vi "Probe.vi"() -> ()   [LabVIEW 2020]
uses:
  source/PV Data/NT Base/NT Base.lvclass
  source/Client/Subscription/Subscription.lvclass
  source/Client/Client/Client.lvclass
  source/PV Data/Is Probeable/Is Probeable.lvclass
  source/Client/Subscription/Next Value - NT.vi
panel:
  in  "Search":bool
  in  "PV name":string
  in  "stop":bool
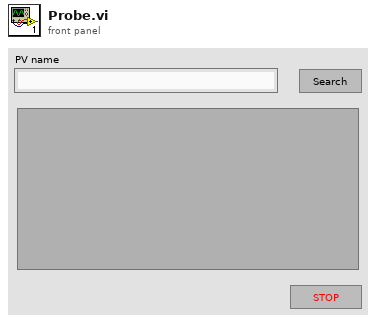
[diagram p1: front panel]
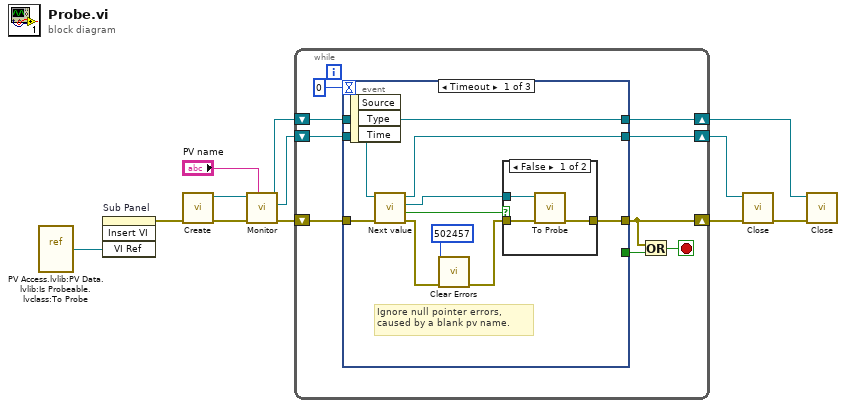
[diagram p0: block diagram]
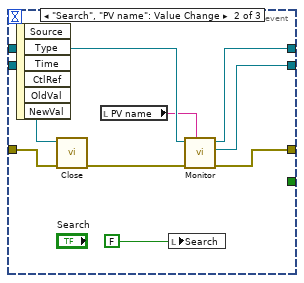
[diagram p3: hidden frame]
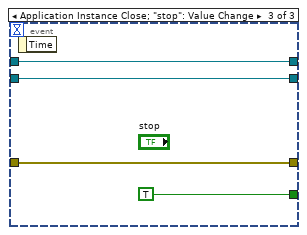
[diagram p4: hidden frame]
diagram:
  n1 = vi-ref "PV Access.lvlib:PV Data.lvlib:Is Probeable.lvclass:To Probe.vi"() -> (w7:refnum<vi>)
  n2 = invoke on="Sub Panel" class="SubPnl" method="Insert VI"("VI Ref"=w7) -> (error out=w8:errorcluster)  [unwired: 3 in, 3 out]
  n3 = call "Create.vi"("error in (no error)"=w8) -> ("error out"=w6:errorcluster, "Client out"=w5:refnum<class "Client.lvclass">)  [unwired: 9 in]
  n4 = call "Monitor.vi"("PV name"="PV name", "error in"=w6, "Client in"=w5) -> ("error out"=w3:errorcluster, "subscription"=w2:refnum<class "Subscription.lvclass">, "Client out"=w4:refnum<class "Client.lvclass">)  [unwired: 6 in]
  n5 = while {
    shift-right: [w19] -> w12
    shift-left: w4 -> [w20]
    shift-right: [w16] -> w11
    shift-left: w3 -> [w21]
    shift-right: [w15] -> w9
    shift-left: w2 -> [w14]
    stop <- w17 stop-if-true
    n6 = event shown="[0] Timeout" {
      selector: _ -> [_ _ _]
      dyn-events: _ -> [_ _ _]
      timeout: 0 -> [_ _ _]
      tunnel: w21 -> [w30 w40 w47]
      tunnel: w20 -> [w31 w41 w46]
      tunnel: [w29 w36 w47] -> w16
      tunnel: [w31 w44 w46] -> w19
      tunnel: [_ _ TRUE] -> w18
      tunnel: [w28 w43 w45] -> w15
      tunnel: w14 -> [w27 w42 w45]
      event Timeout {
        # "Ignore null pointer errors, caused by a blank pv name."
        n7 = event-data() -> ()  [unwired: 1 in, 3 out]
        n8 = call-poly "Next value.vi"("error in (no error)"=w30, "Subscription in"=w27) -> ("error out"=w26:errorcluster, "timed out?"=w22:bool, "value"=w23:refnum<class "NT Base.lvclass">, "Subscription out"=w28:refnum<class "Subscription.lvclass">)  [unwired: 5 in, 1 out]
        n9 = call <vilib>:"Clear Errors.vi"("error in (no error)"=w26, "specific error code to clear (0: all)"=502457) -> ("error out"=w25:errorcluster)  [unwired: 4 in, 1 out]
        n10 = case shown="False" w22 {
          tunnel: [w34 w35] -> w29
          tunnel: w25 -> [w33 w35]
          tunnel: w23 -> [w32 _]
          frame False {
            n11 = call-dynamic "To Probe.vi"("error in (no error)"=w33, "Is Probeable in"=w32) -> ("error out"=w34:errorcluster)  [unwired: 7 in, 2 out]
          }
          frame True {
          }
        }
      }
      event "Search", "PV name": Value Change {
        n12 = event-data() -> ()  [unwired: 1 in, 6 out]
        n13 = call-dynamic "Close.vi"("error in (no error)"=w40, "Subscription in"=w42) -> ("error out"=w38:errorcluster)  [unwired: 9 in]
        n14 = local read "PV name"() -> (w37:string)
        n15 = local write "Search"(FALSE ("Search")) -> ()
        n16 = call "Monitor.vi"("PV name"=w37, "error in"=w38, "Client in"=w41) -> ("error out"=w36:errorcluster, "subscription"=w43:refnum<class "Subscription.lvclass">, "Client out"=w44:refnum<class "Client.lvclass">)  [unwired: 6 in]
      }
      event Application Instance Close; "stop": Value Change {
        n17 = event-data() -> ()  [unwired: 1 in, 1 out]
      }
    }
    n18 = Or(x=w16, y=w18) -> (x .or. y?=w17:bool)
  }
  n19 = call-dynamic "Close.vi"("error in (no error)"=w11, "Subscription in"=w9) -> ("error out"=w10:errorcluster)  [unwired: 9 in]
  n20 = call "Close.vi"("error in (no error)"=w10, "Client in"=w12) -> ()  [unwired: 9 in, 1 out]
